vi "Strip Tag in Tag Value Pair.vi"(11 "Tag:Value":string="Tag : Value") -> (3 "Value":string="Value")   [LabVIEW 2017, in "API String Arguments Support.lvlib"]
uses:
  API String Arguments Support.lvlib
  <userlib>/_NEVSTOP/Communicable State Machine(CSM)/Communicable State Machine.lvlib
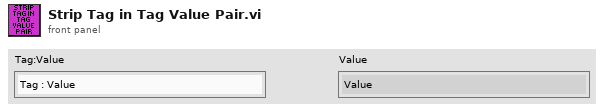
[diagram p1: front panel]
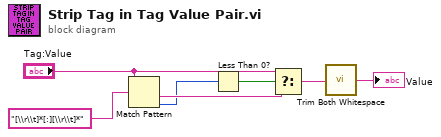
[diagram p0: block diagram]
diagram:
  n1 = Match Pattern(string="Tag:Value", regular expression="[\\r\\t]*[:][\\r\\t]*") -> (after substring=w6:string, offset past match=w4:i32)  [unwired: 1 in, 2 out]
  n2 = Less Than 0?(x=w4) -> (x < 0?=w3:bool)
  n3 = Select(t="Tag:Value", s=w3, f=w6) -> (s? t:f=w2:string)
  n4 = call <userlib>:"Trim Both Whitespace.vi"("string"=w2) -> ("trimmed string"=→"Value":string)  [unwired: 1 in]
